vi "GetControlRefByArray.vi"(0 "VI Reference In":refnum<vi>, 7 "Control Path":string[](array[string]), 11 "error In":errorcluster) -> (4 "VI Reference Out":refnum<vi>, 8 "Ctl Refnum":refnum<vi>, 15 "error out":errorcluster)   [LabVIEW 2016, in "Drona.lvlib" / "GetControlRef.lvlib"]
doc: "Gives the reference of control which is specified.\n\nThe path of the control should be given in the successive index of the array"
uses:
  GetControlRef.lvlib
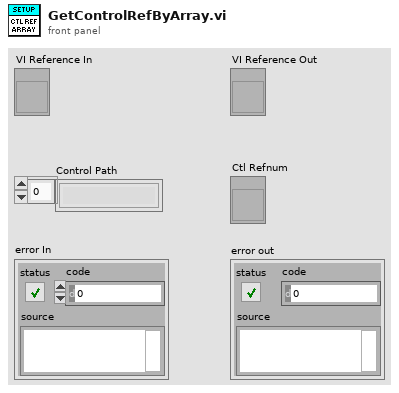
[diagram p1: front panel]
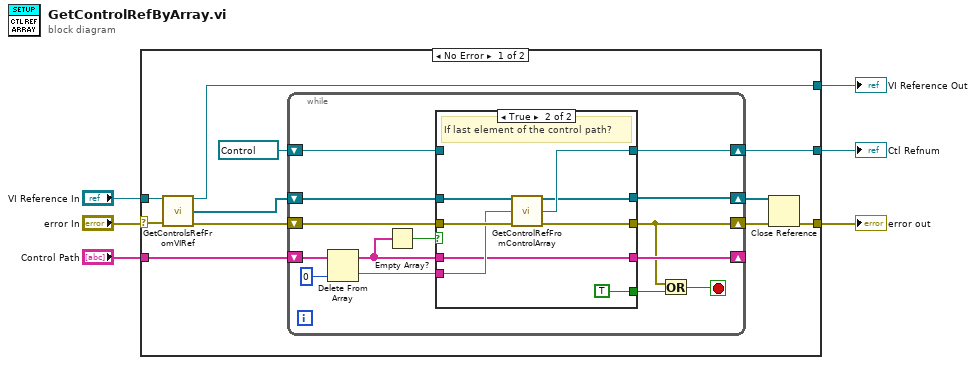
[diagram p0: block diagram]
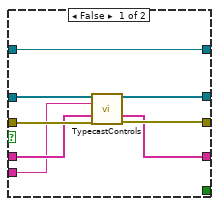
[diagram p2: hidden frame]
diagram:
  n1 = case shown="No Error" "error In" {
    selector: "error In" -> [w10 w49]
    tunnel: "Control Path" -> [w16 _]
    tunnel: [w9 w49] -> w5
    tunnel: [w13 _] -> w4
    tunnel: "VI Reference In" -> [w11 w48]
    tunnel: [w8 w48] -> w1
    frame No Error {
      n2 = call "GetControlsRefFromVIRef.vi"("VI Reference In"=w11, "Error In"=w10) -> ("VI Reference Out"=w8:refnum<vi>, "Controls[]"=w15:refnum<vi>[], "Error Out"=w12:errorcluster)  [unwired: 11 in]
      n3 = while {
        shift-right: [w19] -> w17
        shift-left: w12 -> [w29]
        shift-right: [w26] -> w14
        shift-left: w15 -> [w27]
        shift-right: [w22] -> w13
        shift-left: refnum<vi> refnum ("Target Control") -> [w25]
        shift-right: [w24] -> _
        shift-left: w16 -> [w28]
        stop <- w18 stop-if-true
        n4 = Delete From Array(array=w28, index=0) -> (deleted portion=w30:string, array with subset deleted=w23:string[])  [unwired: 1 in]
        n5 = Empty Array?(array=w23) -> (empty?=w31:bool)
        n6 = case shown="True" w31 {
          tunnel: w27 -> [w39 w45]
          tunnel: w30 -> [w32 w46]
          tunnel: [w35 w43] -> w22
          tunnel: w29 -> [w38 w47]
          tunnel: [w36 w44] -> w19
          tunnel: [w37 w42] -> w26
          tunnel: w25 -> [w35 _]
          tunnel: [_ TRUE] -> w20
          tunnel: w23 -> [w34 w40]
          tunnel: [w33 w40] -> w24
          frame False {
            n7 = call "TypecastControls.vi"("Controls[]"=w39, "Control Name"=w32, "Control Path In"=w34, "error In"=w38) -> ("Sub Controls[]"=w37:refnum<vi>[], "Control Path Out"=w33:string[], "error out"=w36:errorcluster)  [unwired: 9 in]
          }
          frame True {
            # "If last element of the control path?"
            n8 = call "GetControlRefFromControlArray.vi"("Controls[]"=w45, "Control Path"=w46, "error In"=w47) -> ("Remaining Controls[]"=w42:refnum<vi>[], "Target Control"=w43:refnum<vi>, "error out"=w44:errorcluster)  [unwired: 10 in]
          }
        }
        n9 = Or(x=w19, y=w20) -> (x .or. y?=w18:bool)
      }
      n10 = Close Reference(reference=w14, error in (no error)=w17) -> (error out=w9:errorcluster)
    }
    frame Error {
    }
  }
  "Ctl Refnum" <- w4
  "error out" <- w5
  "VI Reference Out" <- w1
